vi "Create Data Channel - Array - Format.vi"(8 "error in (no error)":errorcluster, 9 "settings":T2, 10 "channel name":string, 11 "response refnum in":T1 format="%.0x") -> (0 "error out":errorcluster, 1 "channel refnums":T1[](array[typedef]) format="%.0x", 2 "array refnum":T1=18446744073709551615 format="%.0x", 3 "response refnum out":T1 format="%.0x")   [LabVIEW 2020, in "Instrument Addon Scripting API.lvlib"]
doc: "Creates a new Data Channel Array under the specified response."
uses:
  Instrument Addon Scripting API.lvlib
  <vilib>/NI VeriStand/Custom Device API/Custom Device Item Ref.ctl
  TypeDefs/Array Format Settings.ctl
  TypeDefs/Array Element.ctl
  Shared Directory/Data Parameters.ctl
  Shared Directory/Protocol Data Type.ctl
  Shared Directory/Data Channel Type.ctl
  Shared Directory/Type Cast Type.ctl
  Shared Directory/Endian.ctl
  Shared Directory/Instrument Addon Shared.lvlib
  <vilib>/NI VeriStand/Custom Device API/Custom Device API.lvlib
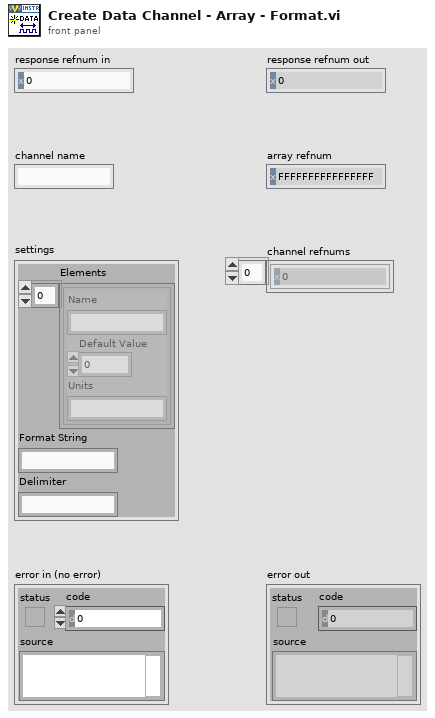
[diagram p1: front panel]
types:
  T1 = typedef "Custom Device API.lvlib/Custom Device Item Ref.ctl" = u64
  T2 = typedef "Instrument Addon Scripting API.lvlib/Array Format Settings.ctl" = cluster{"Elements":T3[], "Format String":string, "Delimiter":string}
  T3 = typedef "Instrument Addon Scripting API.lvlib/Array Element.ctl" = cluster{"Name":string, "Default Value":dbl, "Units":string}
  T4 = typedef "Instrument Addon Shared.lvlib/Data Channel Type.ctl" = enum16{"Format", "Comparison", "Type Cast", "Enumerated List"}
  T5 = typedef "Instrument Addon Shared.lvlib/Protocol Data Type.ctl" = enum16{"Single Channel", "Array"}
  T6 = typedef "Instrument Addon Shared.lvlib/Data Parameters.ctl" = cluster{"Data Type":T5, "Channel Type":T4, "Format String":string, "Expected String":string, "Type":T7, "List":string[], "Delimiter":string, "Endian":T8}
  T7 = typedef "Instrument Addon Shared.lvlib/Type Cast Type.ctl" = enum16{"DBL", "SGL", "U64", "U32", "U16", "U8", "I64", "I32", "I16", "I8"}
  T8 = typedef "Instrument Addon Shared.lvlib/Endian.ctl" = enum16{"Native", "Little", "Big"}
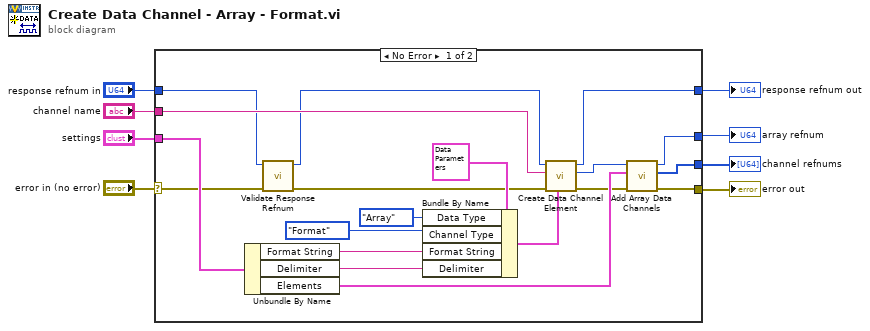
[diagram p0: block diagram]
diagram:
  n1 = case shown="No Error" "error in (no error)" {
    selector: "error in (no error)" -> [w12 w29]
    tunnel: [w22 w29] -> w8
    tunnel: [w14 w28] -> w7
    tunnel: "channel name" -> [w19 _]
    tunnel: "response refnum in" -> [w10 w28]
    tunnel: "settings" -> [w21 _]
    tunnel: [w15 _] -> w2
    tunnel: [w13 _] -> w1
    frame No Error {
      n2 = Unbundle By Name(w21) -> ("Format String"=w24:string, "Delimiter"=w23:string, "Elements"=w20:T3[])
      n3 = call "Validate Response Refnum.vi"("error in (no error)"=w12, "response refnum in"=w10) -> ("error out"=w11:errorcluster, "response refnum out"=w9:u64)  [unwired: 8 in]
      n4 = Bundle By Name(cluster=T6 {"Data Type"=enum."Array", "Channel Type"=enum."Format", "Format String"="%.3g", "Expected String"="", "Type"=enum."SGL", "List"=[], "Delimiter"=",", "Endian"=enum."Native"} ("Settings"), "Data Type"=Protocol_Data_Type."Array", "Channel Type"=Data_Channel_Type."Format", "Format String"=w24, "Delimiter"=w23) -> (w18:T6)
      n5 = call "Create Data Channel Element.vi"("Data Channel Parameters"=w18, "Error In"=w11, "Name"=w19, "Refnum In"=w9) -> ("Error Out"=w16:errorcluster, "Channel Refnum"=w17:T1, "Refnum Out"=w14:T1)  [unwired: 5 in]
      n6 = call "Add Array Data Channels.vi"("error in (no error)"=w16, "array elements"=w20, "section refnum in"=w17) -> ("error out"=w22:errorcluster, "channel refs"=w15:T1[], "array refnum"=w13:T1)  [unwired: 6 in]
    }
    frame Error {
    }
  }
  "error out" <- w8
  "response refnum out" <- w7
  "channel refnums" <- w2
  "array refnum" <- w1
